vi "Load Dut.vi"(8 "error in (no error)":errorcluster, 9 "path in":path=path "D:/Cobham_QCA9984/DUT/dut_control/QCA_DUT_Func.dll", 10 "Bin_file":string, 11 "chip_select":i32) -> (0 "error out":errorcluster, 2 "Bin_file out":string, 3 "return type":u8)   [LabVIEW 2015, in "QCA_DUT_Func.lvlib"]
doc: "DLL_QMSL_AEROFLEX bool _stdcall LoadDut(int chip_select, char Bin_file[100]);"
uses:
  QCA_DUT_Func.lvlib
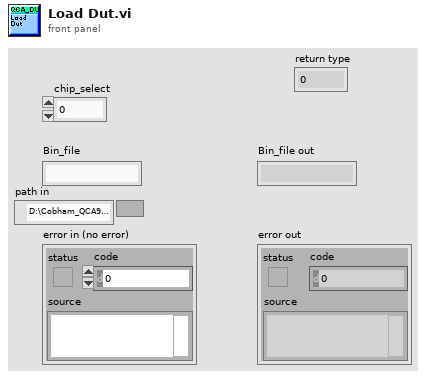
[diagram p1: front panel]
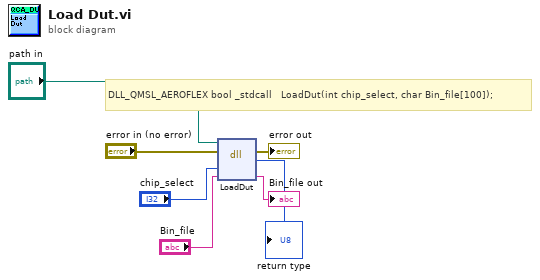
[diagram p0: block diagram]
diagram:
  # "DLL_QMSL_AEROFLEX bool _stdcall   LoadDut(int chip_select, char Bin_file[100]);"
  n1 = dll-call lib="D:/4-Up-WLAN-Test-System/DUT Control/DUT/dut_control/QCA_DUT_Func.dll" fn="LoadDut"(path in="path in", error in="error in (no error)", "chip_select"="chip_select", "Bin_file"="Bin_file") -> (error out=→"error out":errorcluster, "return type"=→"return type":i32, "Bin_file"=→"Bin_file out":string)  [unwired: 2 in, 1 out]
